vi "ESP_Upload_Long.vi"(0 "Motion Settings In":T1={"No Motion?"=FALSE, "Motion System"=enum."NI 735x", "Motion Bd ID"=1, "Motion Profile"="SMAC1", "# Axis"=1, "Reverse Z axis?"=TRUE, "SMAC Axis"=0, "scan pair"=enum."y-(x) scan", "RT fps"=6.0, "Steps per mm"=[1000, 1000, 1000, 1000], "Motor Parameters"={"velocity ct/s"=[10000.0, 10000.0, 10000.0, 50000.0], "accel ct/s^2"=[50000.0, 50000.0, 50000.0, 200000.0]}, "One Way Scan"=FALSE, "Reverse One Way Scan"=FALSE, "Global Position (mm)"=[], "Plane"=0, "Distance between\nscan lines (um)"=0.0, "Distance between\nscan planes (um)"=0.0, "number of scan planes"=1, "Total steps in line"=0, "Xtra plane\ndistance  (um)"=100, "Xtra planes "=1, "Add Axis"=FALSE, "overshoot cts"=200, "BKPT Shift"=0, "Scan Start Time (ms)"=0, "ESP VISA"="GPIB::1::INSTR", "3rd Axis"=1, "GL Ref Out"=refnum, "Galil Address"=""} {"3rd Axis" items=["x", "y", "z", "w"]; "Xtra planes" min=1; "Xtra plane\ndistance  (um)" min=0; "Distance between\nscan planes (um)" format="%.2f"; "Distance between\nscan lines (um)" format="%.2f"; "SMAC Axis" items=["None"=0, "Axis 1"=1, "Axis 2"=2, "Axis 3"=3, "Axis 4"=4, "Axis 5"=5, "Axis 6"=6, "Axis 7"=7, "Axis 8"=8, "Vector Space 1"=17, "Vector Space 2"=18, "Vector Space 3"=19, "Vector Space 4"=20]; "Motion Bd ID" min=1 max=32 step=1}, 1 "Axis":i32=1 min=1 max=4, 2 "Purge?":bool, 3 "lines per scan":i32=128, 5 "Program#":i32=2, 9 "Reverse ?":bool, 11 "error in":errorcluster, 14 "Offset":i32) -> (4 "VISA resource name out":refnum<visa-resource-name>, 15 "error out":errorcluster)   [LabVIEW 2022 SP3]
uses:
  NI_controller/-NI_MotionRoutines/MotionParameters.ctl
  NI_controller/-NI_MotionRoutines/MotionSys.ctl
  -MotionRoutines/ScanAxis.ctl
  -MotionRoutines/3rdAxis.ctl
  <instrlib>/Newport ESP301/Newport ESP301.lvlib
panel:
  # "1-D and 2-D B scan settings"
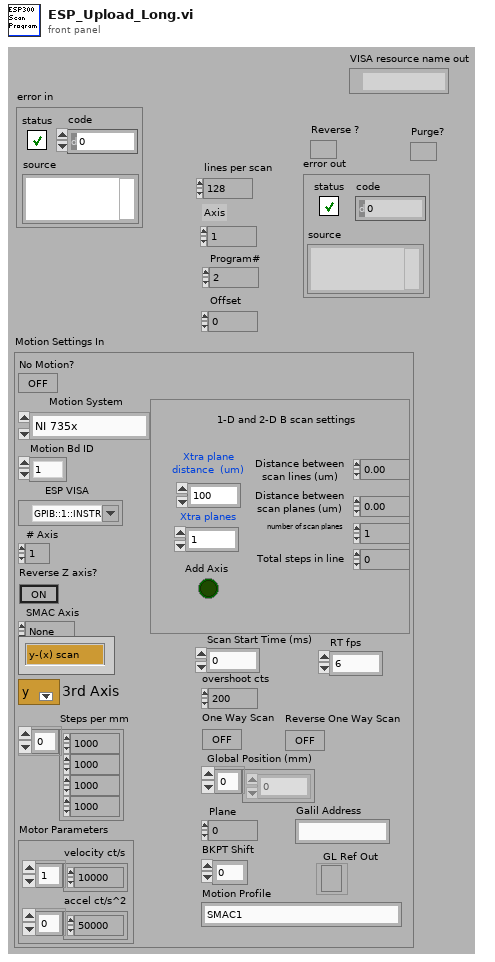
[diagram p1: front panel]
types:
  T1 = typedef "MotionParameters.ctl" = cluster{"No Motion?":bool, "Motion System":T2, "Motion Bd ID":u8, "Motion Profile":string, "# Axis":i8, "Reverse Z axis?":bool, "SMAC Axis":u16, "scan pair":T3, "RT fps":sgl, "Steps per mm":i32[], "Motor Parameters":cluster{"velocity ct/s":dbl[], "accel ct/s^2":dbl[]}, "One Way Scan":bool, "Reverse One Way Scan":bool, "Global Position (mm)":dbl[], "Plane":i32, "Distance between\nscan lines (um)":sgl, "Distance between\nscan planes (um)":sgl, "number of scan planes":i32, "Total steps in line":i32, "Xtra plane\ndistance  (um)":i32, "Xtra planes ":i32, "Add Axis":bool, "overshoot cts":i32, "BKPT Shift":i32, "Scan Start Time (ms)":u32, "ESP VISA":refnum<visa-resource-name>, "3rd Axis":T4, "GL Ref Out":refnum<k7>, "Galil Address":string}
  T2 = typedef "MotionSys.ctl" = enum16{"MM3000", "NI 735x", "Newport ESP", "No Motion Card", "Galil"}
  T3 = typedef "ScanAxis.ctl" = enum16{"y-(x) scan", "x-(y) scan", "z-(x) scan", "z-(y) scan", "y-(z) scan", "x-(z) scan", "w-(x) scan", "w-(y) scan", "w-(z) scan", "x-(w) scan", "y-(w) scan", "z-(w) scan"}
  T4 = typedef "3rdAxis.ctl" = u16
  T5 = cluster{"Port A bit-0 at logic level":bool, "Port A bit-1 at logic level":bool, "Port A bit-2 at logic level ":bool, "Port A bit-3 at logic level":bool, "Port A bit-4 at logic level":bool, "Port A bit-5 at logic level ":bool, "Port A bit-6 at logic level ":bool, "Port A bit-7 at logic level ":bool, "Port B bit-0 at logic level":bool, "Port B bit-1 at logic level":bool, "Port B bit-2 at logic level ":bool, "Port B bit-3 at logic level":bool, "Port B bit-4 at logic level":bool, "Port B bit-5 at logic level ":bool, "Port B bit-6 at logic level ":bool, "Port B bit-7 at logic level ":bool}
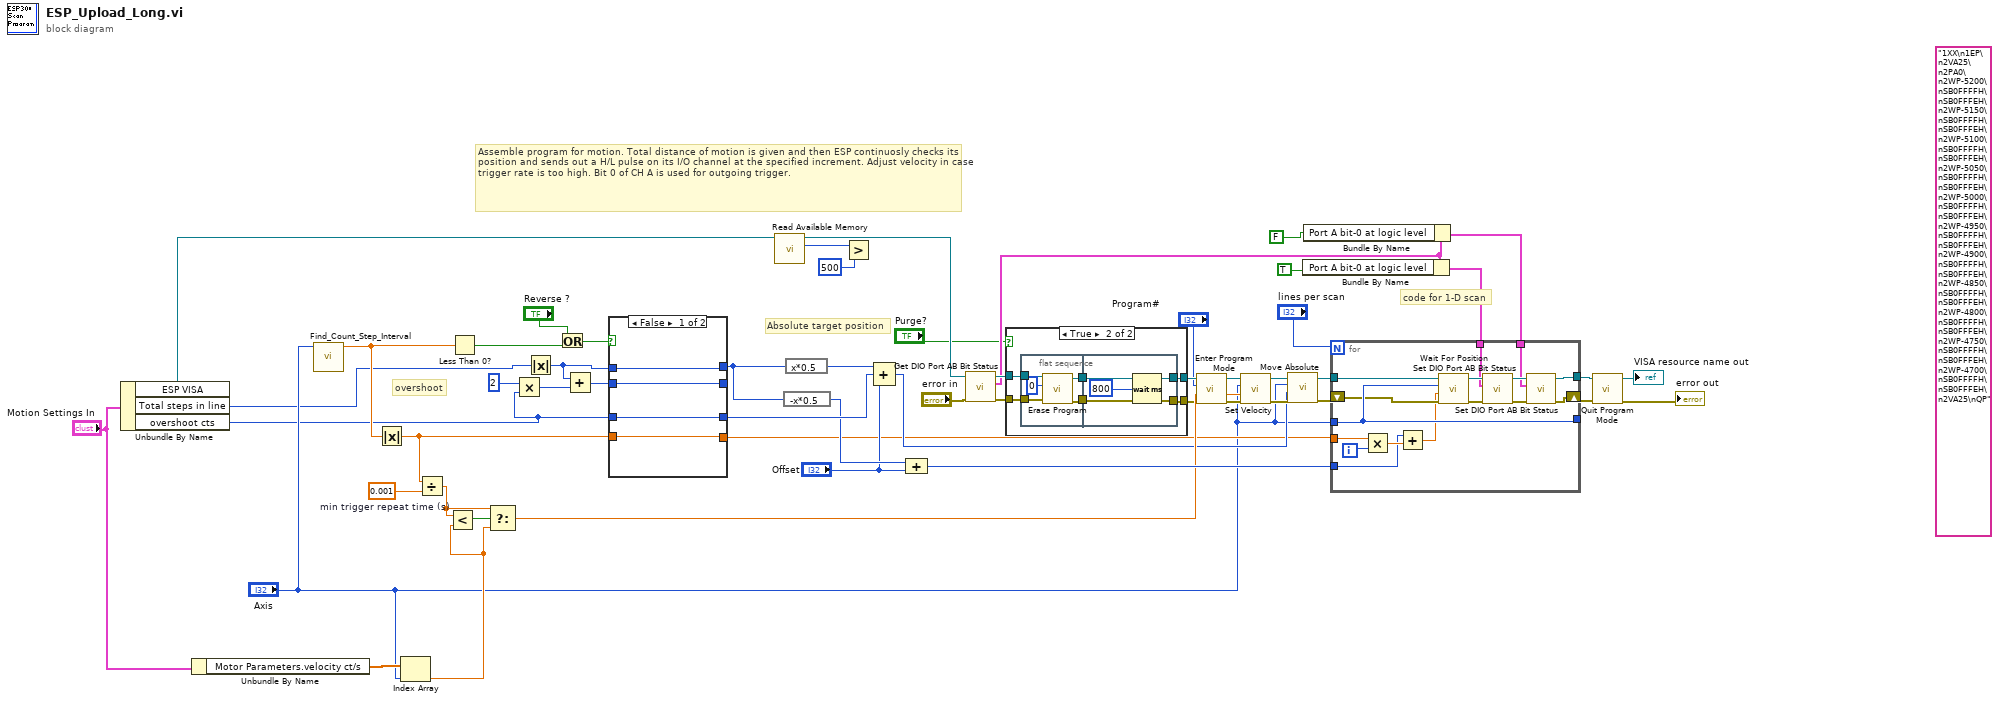
[diagram p0: block diagram]
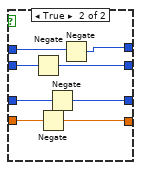
[diagram p3: hidden frame]
diagram:
  (unwired) "1XX\n1EP\n2VA25\n2PA0\n2WP-5200\nSB0FFFFH\nSB0FFFEH\n2WP-5150\nSB0FFFFH\nSB0FFFEH\n2WP-5100\nSB0FFFFH\nSB0FFFEH\n2WP-5050\nSB0FFFFH\nSB0FFFEH\n2WP-5000\nSB0FFFFH\nSB0FFFEH\n2WP-4950\nSB0FFFFH\nSB0FFFEH\n2WP-4900\nSB0FFFFH\nSB0FFFEH\n2WP-4850\nSB0FFFFH\nSB0FFFEH\n2WP-4800\nSB0FFFFH\nSB0FFFEH\n2WP-4750\nSB0FFFFH\nSB0FFFEH\n2WP-4700\nSB0FFFFH\nSB0FFFEH\n2VA25\nQP" ("Output String")
  w39 = 0.001  # min trigger repeat time (s)
  # "code for 1-D scan"
  # "Absolute target position"
  # "overshoot"
  # "Assemble program for motion. Total distance of motion is given and then ESP continuosly checks its position and sends out a H/L pulse on its I/O channel at the specified increment. Adjust velocity in case trigger rate is too high. Bit 0 of CH A is used for outgoing trigger."
  n1 = Unbundle By Name("Motion Settings In") -> ("ESP VISA"=w2:refnum<visa-resource-name>, "Total steps in line"=w1:i32, "overshoot cts"=w3:i32)
  n2 = Unbundle By Name("Motion Settings In") -> ("Motor Parameters.velocity ct/s"=w8:dbl[])
  n3 = call "Find_Count_Step_Interval.vi"("Axis"="Axis") -> ("BP Interval"=w6:dbl)  [unwired: 9 in, 1 out]
  n4 = Absolute Value(x=w6) -> (abs(x)=w47:dbl)
  n5 = Index Array(array=w8, index="Axis") -> (element=w7:dbl)
  n6 = Divide(x=w47, y=w39) -> (x/y=w40:dbl)
  n7 = Less?(x=w40, y=w7) -> (x < y?=w41:bool)
  n8 = Less Than 0?(x=w6) -> (x < 0?=w53:bool)
  n9 = Select(t=w40, s=w41, f=w7) -> (s? t:f=w26:dbl)
  n10 = Multiply(x=2, y=w3) -> (x*y=w48:i32)
  n11 = Absolute Value(x=w1) -> (abs(x)=w50:i32)
  n12 = Or(x="Reverse ?", y=w53) -> (x .or. y?=w51:bool)
  n13 = Add(x=w50, y=w48) -> (x+y=w46:i32)
  n14 = case shown="False" w51 {
    tunnel: w46 -> [w58 w66]
    tunnel: [w58 w65] -> _
    tunnel: [w57 w63] -> w43
    tunnel: w3 -> [w57 w64]
    tunnel: w47 -> [w56 w62]
    tunnel: [w56 w61] -> w9
    tunnel: [w55 w59] -> w45
    tunnel: w50 -> [w55 w60]
    frame False {
    }
    frame True {
      n15 = Negate(x=w66) -> (-x=w65:i32)
      n16 = Negate(x=w62) -> (-x=w61:dbl)
      n17 = Negate(x=w64) -> (-x=w63:i32)
      n18 = Negate(x=w60) -> (-x=w59:i32)
    }
  }
  n19 = call <instrlib>:"Read Available Memory.vi"("VISA resource name"=w2) -> ("Available Storage Space"=w14:i32, "VISA resource name out"=w13:refnum<visa-resource-name>)  [unwired: 4 in, 1 out]
  n20 = expression code="-x*0.5"(w45) -> (w42:i32)
  n21 = expression code="x*0.5"(w45) -> (w44:i32)
  n22 = Greater?(x=w14, y=500) -> ()  [unwired: 1 out]
  n23 = Compound Arithmetic op=ADD(w44, w43, "Offset") -> (w25:i32)
  n24 = Compound Arithmetic op=ADD(w42, "Offset") -> (w38:i32)
  n25 = call <instrlib>:"Get DIO Port AB Bit Status.vi"("error in (no error)"="error in", "VISA resource name"=w13) -> ("error out"=w28:errorcluster, "DIO Port A status"=w23:T5, "VISA resource name out"=w29:refnum<visa-resource-name>)  [unwired: 3 in]
  n26 = case shown="True" "Purge?" {
    tunnel: [w68 w73] -> w34
    tunnel: w29 -> [w68 w72]
    tunnel: w28 -> [w67 w71]
    tunnel: [w67 w74] -> w11
    frame False {
    }
    frame True {
      n27 = flat-sequence {
        tunnel: w72 -> [w77]
        tunnel: w71 -> [w76]
        tunnel: [w79] -> w70
        tunnel: [w78] -> w69
        tunnel: [w81] -> w73
        tunnel: [w82] -> w74
        tunnel: w70 -> [w82]
        tunnel: w69 -> [w81]
        frame #0 {
          n28 = call <instrlib>:"Erase Program.vi"("error in (no error)"=w76, "Program # (1)"=0, "VISA resource name"=w77) -> ("error out"=w79:errorcluster, "VISA resource name out"=w78:refnum<visa-resource-name>)  [unwired: 3 in]
        }
        frame #1 {
          n29 = Wait (ms)(milliseconds to wait=800) -> ()  [unwired: 1 out]
        }
      }
    }
  }
  n30 = call <instrlib>:"Enter Program Mode.vi"("error in (no error)"=w11, "Program Number (1)"="Program#", "VISA resource name"=w34) -> ("error out"=w33:errorcluster, "VISA resource name out"=w32:refnum<visa-resource-name>)  [unwired: 3 in]
  n31 = call <instrlib>:"Set Velocity.vi"("error in (no error)"=w33, "Velocity (units/s)"=w26, "Axis (1)"="Axis", "VISA resource name"=w32) -> ("error out"=w31:errorcluster, "VISA resource name out"=w30:refnum<visa-resource-name>)  [unwired: 2 in]
  n32 = call <instrlib>:"Move Absolute.vi"("error in (no error)"=w31, "Position (0 units)"=w25, "Axis (1)"="Axis", "VISA resource name"=w30) -> ("error out"=w17:errorcluster, "VISA resource name out"=w24:refnum<visa-resource-name>)  [unwired: 2 in]
  n33 = Bundle By Name(cluster=w23, "Port A bit-0 at logic level"=TRUE) -> (w22:T5)
  n34 = Bundle By Name(cluster=w23, "Port A bit-0 at logic level"=FALSE) -> (w21:T5)
  n35 = for {
    N: "lines per scan" -> [_]
    tunnel: w9 -> [w96]
    tunnel: w38 -> [w95]
    tunnel: "Axis" -> [w86]
    tunnel: w24 -> [w94]
    tunnel: w22 -> [w89]
    tunnel: w21 -> [w88]
    tunnel: [w87] -> w16
    tunnel: [w86] -> _
    shift-right: [w85] -> w15
    shift-left: w17 -> [w84]
    i -> [w98]
    n36 = Multiply(x=w96, y=w98) -> (x*y=w97:dbl)
    n37 = Add(x=w95, y=w97) -> (x+y=w83:dbl)
    n38 = call <instrlib>:"Wait For Position.vi"("error in (no error)"=w84, "Position (0 units)"=w83, "Axis (1)"=w86, "VISA resource name"=w94) -> ("error out"=w92:errorcluster, "VISA resource name out"=w93:refnum<visa-resource-name>)  [unwired: 2 in]
    n39 = call <instrlib>:"Set DIO Port AB Bit Status.vi"("error in (no error)"=w92, "DIO Port status"=w89, "VISA resource name"=w93) -> ("error out"=w90:errorcluster, "VISA resource name out"=w91:refnum<visa-resource-name>)  [unwired: 3 in]
    n40 = call <instrlib>:"Set DIO Port AB Bit Status.vi"("error in (no error)"=w90, "DIO Port status"=w88, "VISA resource name"=w91) -> ("error out"=w85:errorcluster, "VISA resource name out"=w87:refnum<visa-resource-name>)  [unwired: 3 in]
  }
  n41 = call <instrlib>:"Quit Program Mode.vi"("error in (no error)"=w15, "VISA resource name"=w16) -> ("error out"=→"error out":errorcluster, "VISA resource name out"=→"VISA resource name out":refnum<visa-resource-name>)  [unwired: 4 in]
